vi "Auton Drive Gyro & Encoder Straight at Angle Slow.vi"(8 "Angle Setpoint":dbl, 10 "Distance Set Point":dbl=-70.0) -> (3 "At Destination?":bool=TRUE)   [LabVIEW 2014]
uses:
  <vilib>/Rock Robotics/WPI/RobotDrive/WPI_RobotDriveGetSetRefNum.vi
  <vilib>/addons/control/pid/pid.llb/PID (DBL).vi
  <vilib>/Rock Robotics/Network Tables/SD Write Number.vi
  <vilib>/Rock Robotics/WPI/RobotDrive/WPI_RobotDriveArcadeDrive_Standard(NoSaturation).vi
  <vilib>/addons/control/pid/NI_PID_pid.lvlib
panel:
  out "In range encoder?":bool=TRUE
  out "Y Value Forward/Rev":dbl=-0.2579279103479475 format="%.2f"
  in  "Gyro Gains":T1={"proportional gain (Kc)"=0.033, "integral time (Ti, min)"=0.0, "derivative time (Td, min)"=0.0} {"derivative time (Td, min)" format="%.3f"; "integral time (Ti, min)" format="%.3f"; "proportional gain (Kc)" format="%.3f"}
  in  "Gyro Range":cluster{"output high":dbl, "output low":dbl}={"output high"=0.65, "output low"=-0.65} {"output low" format="%.2f"; "output high" format="%.2f"}
  out "Gyro Reading":dbl(knob)=4.6535241003020005 scale=-180.0..180.0
  in  "Encoder Destination Range":dbl=2.0
  in  "Gain (VoltsPerDegree/Second)":dbl=0.0066
  in  "Gains":T1={"proportional gain (Kc)"=0.1666, "integral time (Ti, min)"=0.0, "derivative time (Td, min)"=0.0} {"derivative time (Td, min)" format="%.3f"; "integral time (Ti, min)" format="%.3f"; "proportional gain (Kc)" format="%.3f"}
  in  "Range":cluster{"output high":dbl, "output low":dbl}={"output high"=0.6, "output low"=-0.6} {"output low" format="%.2f"; "output high" format="%.2f"}
  # "Field Surface\nHigh .8\nLow -.8"
  # "Robot Room\nHigh .5\nLow -.5"
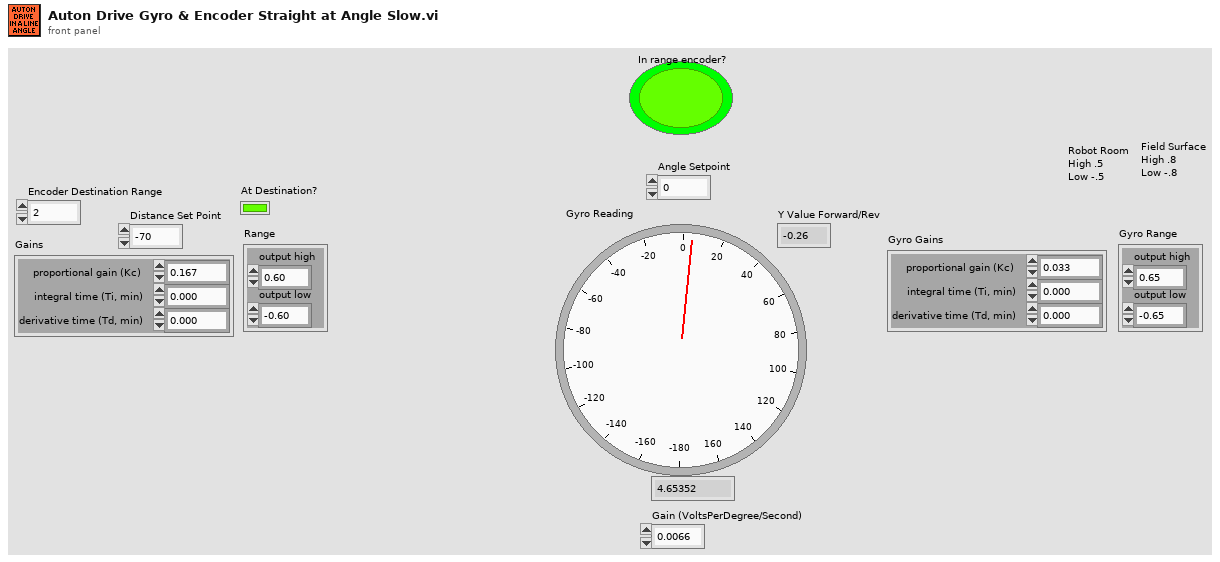
[diagram p1: front panel]
types:
  T1 = cluster{"proportional gain (Kc)":dbl, "integral time (Ti, min)":dbl, "derivative time (Td, min)":dbl}
  T2 = typedef "WPI_GyroDevRef.ctl" = cluster{"DevStatus":errorcluster, "Analog Module":T3, "Analog Channel":T4, "Offset":dbl, "Gain (VoltsPerDegree/Second)":dbl}
  T3 = typedef "FPGA_TypedefAnalogModule.ctl" = enum16{"Controller 1"}
  T4 = typedef "FPGA_AIChannel.ctl" = enum8{"AI 0", "AI 1", "AI 2", "AI 3", "AI MXP 0", "AI MXP 1", "AI MXP 2", "AI MXP 3", "Invalid"}
  T5 = typedef "WPI_EncoderDevRef.ctl" = cluster{"DevStatus":errorcluster, "EncoderIndex":T6, "CounterIndex":T7, "DistancePerCount":dbl, "Decoding Type":T8}
  T6 = typedef "FPGA_EncoderIdx.ctl" = enum8{"Enc 0", "Enc 1", "Enc 2", "Enc 3", "Enc 4", "Enc 5", "Enc 6", "Enc 7", "Invalid"}
  T7 = typedef "FPGA_CounterCtrSystemIndex.ctl" = enum8{"Ctr 0", "Ctr 1", "Ctr 2", "Ctr 3", "Ctr 4", "Ctr 5", "Ctr 6", "Ctr 7", "Invalid"}
  T8 = typedef "WPI_EncoderType.ctl" = enum16{"1x", "2x", "4x"}
  T9 = typedef "WPI_RobotDriveDevRef.ctl" = cluster{"DevStatus":errorcluster, "Motors[]":T10[], "Square Inputs":bool, "Max Output":dbl}
  T10 = typedef "WPI_MotorControlDeviceRef.ctl" = cluster{"DeviceStatus":errorcluster, "Type":T11, "PWM":cluster{"Controller":T12, "PWM Channel":T13, "DeadBand":T14}, "CAN":cluster{"Device Number":u8, "Control Mode":T15, "Semaphore":T16, "Max Vout":dbl, "TalonSRX Control Mode":T17}, "Invert":bool, "TransformRef":T18, "InvTransformRef":T18}
  T11 = typedef "WPI_MotorControlType.ctl" = enum16{"PWM", "CAN", "CANTalonSRX"}
  T12 = typedef "FPGA_TypedefDigitalModule.ctl" = enum16{"Controller 1"}
  T13 = typedef "FPGA_DIOPWMChannel.ctl" = enum8{"PWM 0", "PWM 1", "PWM 2", "PWM 3", "PWM 4", "PWM 5", "PWM 6", "PWM 7", "PWM 8", "PWM 9", "PWM MXP 0", "PWM MXP 1", "PWM MXP 2", "PWM MXP 3", "PWM MXP 4", "PWM MXP 5", "PWM MXP 6", "PWM MXP 7", "PWM MXP 8", "PWM MXP 9", "Invalid"}
  T14 = typedef "WPI_PWMDeadband.ctl" = cluster{"Name":string, "maxPositivePwm":i32, "minPositivePwm":i32, "centerPwm":i32, "maxNegativePwm":i32, "minNegativePwm":i32, "angularRange":u16}
  T15 = typedef "WPI_CANJaguar_ControlMode.ctl" = enum8{"Percent VBus", "Current", "Speed", "Position", "Voltage"}
  T16 = typedef "Semaphore RefNum" = refnum<k1>
  T17 = typedef "WPI_CANTalonSRX_APIControlMode.ctl" = enum8{"Percent VBus", "Speed", "Position", "Slave", "Unchanged / Invalid"}
  T18 = typedef "WPI_PWMTransform_ConPane.ctl" = refnum<vi>
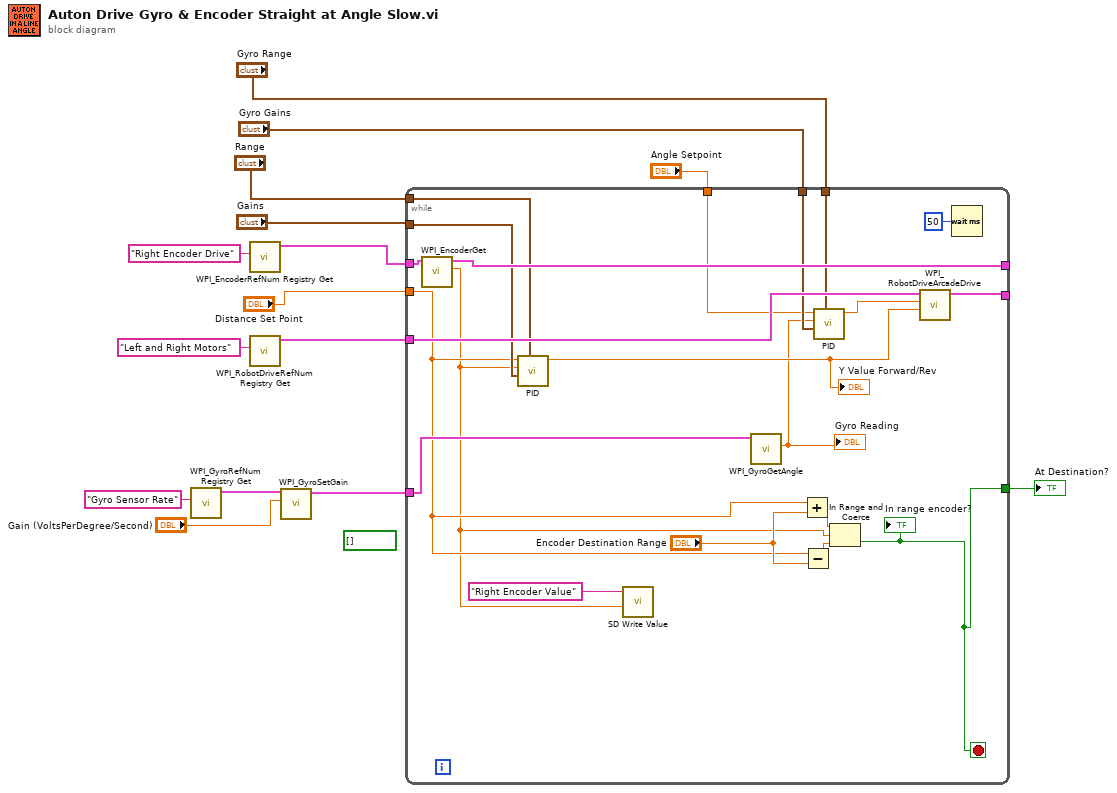
[diagram p0: block diagram]
diagram:
  (unwired) bool[] []
  n1 = call <vilib>:"WPI_GyroRefNum Registry Get.vi"("refnum name"="Gyro Sensor Rate") -> ("GyroDevRef"=w8:T2)  [unwired: 9 in, 1 out]
  n2 = call <vilib>:"WPI_EncoderRefNum Registry Get.vi"("refnum name"="Right Encoder Drive") -> ("EncoderDevRef"=w12:T5)  [unwired: 9 in, 1 out]
  n3 = call <vilib>:"WPI_RobotDriveRefNum Registry Get.vi"("refnum name"="Left and Right Motors") -> ("RobotDriveDevRef"=w14:T9)  [unwired: 9 in, 1 out]
  n4 = call <vilib>:"WPI_GyroSetGain.vi"("Gain (VoltsPerDegree/Second)"="Gain (VoltsPerDegree/Second)", "GyroDevRef"=w8) -> ("GyroDevRef"=w7:T2)  [unwired: 1 in, 8 out]
  n5 = while {
    tunnel: [w35] -> _
    tunnel: [w28] -> _
    tunnel: w14 -> [w27]
    tunnel: w12 -> [w34]
    tunnel: "Distance Set Point" -> [w21]
    tunnel: w7 -> [w30]
    tunnel: "Range" -> [w23]
    tunnel: "Gains" -> [w22]
    tunnel: "Gyro Range" -> [w25]
    tunnel: "Gyro Gains" -> [w24]
    tunnel: "Angle Setpoint" -> [w17]
    tunnel: [w16] -> w1
    stop <- w16 stop-if-true
    n6 = call <vilib>:"WPI_EncoderGet.vi"("EncoderDevRef"=w34) -> ("Distance"=w20:dbl, "EncoderDevRef"=w35:T5)  [unwired: 5 in, 4 out]
    n7 = call-poly <vilib>:"PID.vi"("output range"=w23, "PID gains"=w22, "process variable"=w20, "setpoint"=w21) -> ("output"=w19:dbl)  [unwired: 6 in, 1 out]
    "Y Value Forward/Rev" <- w19
    n8 = call-poly <vilib>:"SD Write Value.vi"("Numeric"=w20, "Name"="Right Encoder Value") -> ()  [unwired: 8 in, 2 out]
    n9 = call <vilib>:"WPI_GyroGetAngle.vi"("GyroDevRef"=w30) -> ("Angle"=w18:dbl)  [unwired: 1 in, 9 out]
    "Gyro Reading" <- w18
    n10 = Add(x=w21, y="Encoder Destination Range") -> (x+y=w33:dbl)
    n11 = Subtract(x=w21, y="Encoder Destination Range") -> (x-y=w32:dbl)
    n12 = call-poly <vilib>:"PID.vi"("output range"=w25, "PID gains"=w24, "process variable"=w18, "setpoint"=w17) -> ("output"=w26:dbl)  [unwired: 6 in, 1 out]
    n13 = In Range and Coerce(upper limit=w33, x=w20, lower limit=w32) -> (In Range?=w16:bool)  [unwired: 1 out]
    "In range encoder?" <- w16
    n14 = call-poly <vilib>:"WPI_RobotDriveArcadeDrive.vi"("Y axis value"=w19, "X axis value"=w26, "RobotDriveDevRef"=w27) -> ("RobotDriveDevRef"=w28:T9)  [unwired: 6 in, 2 out]
    n15 = Wait (ms)(milliseconds to wait=u32 50) -> ()  [unwired: 1 out]
  }
  "At Destination?" <- w1
